vi "Pusher_Client_Close.vi"(8 "ErrIn":errorcluster, 11 "Client in":refnum<class "Client.lvclass">) -> (0 "ErrOut":errorcluster)   [LabVIEW 2009, in "Client.lvclass"]
uses:
  Client.lvclass
  Client.lvclass/Client.ctl
panel:
  out "Client out":refnum<class "Client.lvclass">
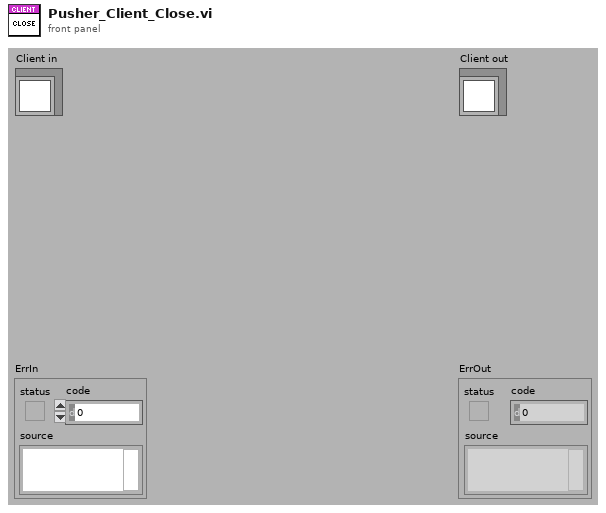
[diagram p1: front panel]
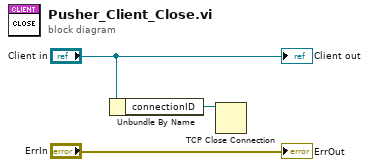
[diagram p0: block diagram]
diagram:
  n1 = Unbundle By Name("Client in") -> ("connectionID"=w1:refnum<k5>)
  n2 = TCP Close Connection(connection ID=w1) -> ()  [unwired: 2 in, 2 out]
  "ErrOut" <- "ErrIn"
  "Client out" <- "Client in"
